vi "Hot_Cold_Accumulated_Gallons.vi"(0 "GEA2 Reference In":refnum<k24>, 1 "GEA Inputs":T2 {"Destination" format="%.0x"; "Source" format="%.0x"}, 11 "Error In":errorcluster, 12 "Repeat Count":i32) -> (2 "Hot Gallons":dbl, 3 "Hot_Cold_Accumulated Gallons":dbl[](array[numeric]), 4 "GEA2 Reference Out":refnum<k24>, 8 "ERD Data Out":T1[](array[typedef]) {"ERD Number" format="%.0x"}, 13 "Cold Gallons":dbl, 14 "Current Tub Gallons":dbl, 15 "Error Out":errorcluster)   [LabVIEW 2016, in "TLMB.lvlib"]
doc: "This vi can be used to read ERD every 1 sec for user selected repeat counts."
uses:
  Projects/TLMB.lvlib
  Q:/Common/DLLs/GEA3/GeaCommunication.dll
  Common/DLLs/GEA3/GeaCommunication.dll
  Common/LabVIEW GEA2 Toolkit/LabVIEW_GEA2_Toolkit.lvlibp/type defs/Source_Destination.ctl
  Common/LabVIEW GEA2 Toolkit/LabVIEW_GEA2_Toolkit.lvlibp/type defs/ERD Read Data Out.ctl
  Common/LabVIEW GEA2 Toolkit/LabVIEW_GEA2_Toolkit.lvlibp/type defs/ERD Read Data In.ctl
  Common/LabVIEW GEA2 Toolkit/LabVIEW_GEA2_Toolkit.lvlibp/type defs/Data Type.ctl
  Common/LabVIEW GEA2 Toolkit/LabVIEW_GEA2_Toolkit.lvlibp
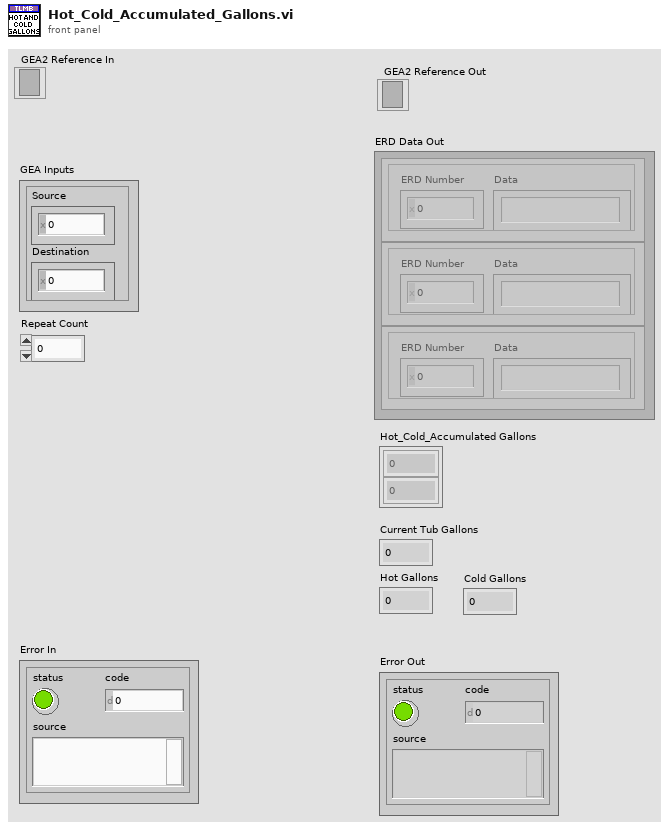
[diagram p1: front panel]
types:
  T1 = typedef "LabVIEW_GEA2_Toolkit.lvlibp/ERD Read Data Out.ctl" = cluster{"ERD Number":u16, "Data":string}
  T2 = typedef "LabVIEW_GEA2_Toolkit.lvlibp/Source_Destination.ctl" = cluster{"Source":u8, "Destination":u8}
  T3 = typedef "LabVIEW_GEA2_Toolkit.lvlibp/ERD Read Data In.ctl" = cluster{"ERD Number":u16, "Data Type":T4}
  T4 = typedef "LabVIEW_GEA2_Toolkit.lvlibp/Data Type.ctl" = enum16{"string", "boolean", "uint8_t", "uint16_t", "uint32_t", "uint64_t", "int8_t", "int16_t", "int32_t", "int64_t"}
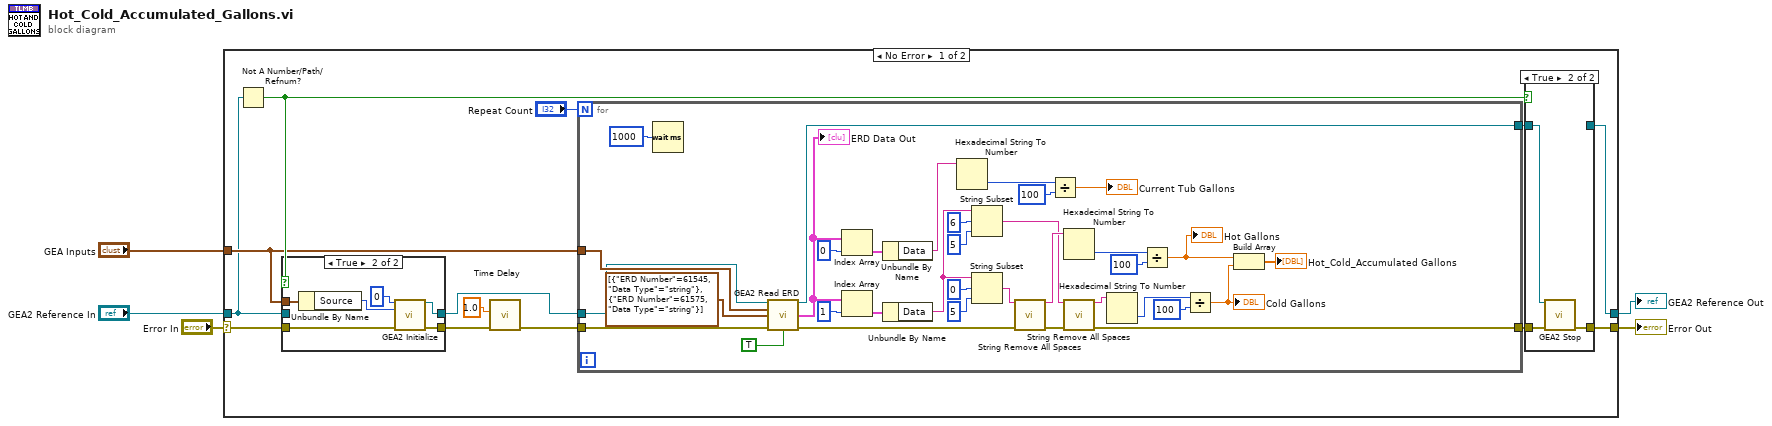
[diagram p0: block diagram]
diagram:
  n1 = case shown="No Error" "Error In" {
    selector: "Error In" -> [w12 w67]
    tunnel: "GEA Inputs" -> [w14 _]
    tunnel: "GEA2 Reference In" -> [w13 w68]
    tunnel: [w11 w68] -> w2
    tunnel: [w10 w67] -> w1
    frame No Error {
      n2 = Not A Number/Path/Refnum?(number/path/refnum=w13) -> (NaN/Path/Refnum?=w15:bool)
      n3 = case shown="True" w15 {
        tunnel: w12 -> [w60 w66]
        tunnel: [w60 w65] -> w8
        tunnel: [w59 w64] -> w9
        tunnel: w14 -> [_ w62]
        tunnel: w13 -> [w59 _]
        frame False {
        }
        frame True {
          n4 = Unbundle By Name(w62) -> ("Source"=w63:u8)
          n5 = call "GEA2 Initialize.vi"("Board Index"=0, "Source Address"=w63, "error in"=w66) -> ("GEA2 Reference Out"=w64:refnum<k24>, "error out"=w65:errorcluster)  [unwired: 10 in, 1 out]
        }
      }
      n6 = call "Time Delay"("error in (no error)"=w8, "Delay Time (s)"=1.0) -> ("error out"=w7:errorcluster)  [unwired: 9 in]
      n7 = for {
        N: "Repeat Count" -> [_]
        tunnel: w14 -> [w53]
        tunnel: [w29] -> w17
        tunnel: [w52] -> w16
        tunnel: w9 -> [w48]
        tunnel: w7 -> [w33]
        n8 = Wait (ms)(milliseconds to wait=u32 1000) -> ()  [unwired: 1 out]
        n9 = call "GEA2 Read ERD.vi"("GEA2 Reference In"=w48, "GEA Inputs"=w53, "Read ERD List"=T3[] [{"ERD Number"=61545, "Data Type"=enum."string"}, {"ERD Number"=61575, "Data Type"=enum."string"}], "Error In"=w33, "Verify ERD Response?"=TRUE) -> ("GEA2 Reference Out"=w52:refnum<k24>, "ERD Data Out"=w38:T1[], "Error Out"=w34:errorcluster)  [unwired: 7 in, 1 out]
        "ERD Data Out" <- w38
        n10 = Index Array(array=w38, index=0) -> (element=w39:T1)
        n11 = Index Array(array=w38, index=1) -> (element=w46:T1)
        n12 = Unbundle By Name(w39) -> ("Data"=w37:string)
        n13 = Unbundle By Name(w46) -> ("Data"=w41:string)
        n14 = Hexadecimal String To Number(string=w37) -> (number=w28:u32)  [unwired: 2 in, 1 out]
        n15 = String Subset(string=w41, offset (0)=6, length (rest)=5 ("length (rest)")) -> (substring=w32:string)
        n16 = String Subset(string=w41, offset (0)=0, length (rest)=5 ("length (rest)")) -> (substring=w36:string)
        n17 = call "String Remove All Spaces.vi"("Input String"=w36, "error in (no error)"=w34) -> ("Spaces Removed"=w35:string, "error out"=w30:errorcluster)  [unwired: 12 in]
        n18 = Divide(x=w28, y=u32 100) -> (x/y=→"Current Tub Gallons":dbl)
        n19 = Hexadecimal String To Number(string=w35) -> (number=w23:u32)  [unwired: 2 in, 1 out]
        n20 = call "String Remove All Spaces.vi"("Input String"=w32, "error in (no error)"=w30) -> ("Spaces Removed"=w31:string, "error out"=w29:errorcluster)  [unwired: 12 in]
        n21 = Hexadecimal String To Number(string=w31) -> (number=w21:u32)  [unwired: 2 in, 1 out]
        n22 = Divide(x=w23, y=u32 100) -> (x/y=w20:dbl)
        "Hot Gallons" <- w20
        n23 = Divide(x=w21, y=u32 100) -> (x/y=w19:dbl)
        "Cold Gallons" <- w19
        n24 = Build Array(w20, w19) -> (→"Hot_Cold_Accumulated Gallons":dbl[])
      }
      n25 = case shown="True" w15 {
        tunnel: w17 -> [w54 w57]
        tunnel: [w54 w56] -> w10
        tunnel: w16 -> [w55 w58]
        tunnel: [w55 _] -> w11
        frame False {
        }
        frame True {
          n26 = call "GEA2 Stop.vi"("GEA2 Reference In"=w58, "Error In"=w57) -> ("Error Out"=w56:errorcluster)  [unwired: 13 in]
        }
      }
    }
    frame Error {
    }
  }
  "GEA2 Reference Out" <- w2
  "Error Out" <- w1
